vi "Edgertronic_SettingDialog.vi"(3 "URL":string="192.168.1.123") -> (1 "Saved Settings:":T4={"Requested Genlock "="20140911165611", "Min Frame Clocks "="20140911165611", "Is Seq Clk Freq "="20140911165611", "Pretrigger Frames "="20140911165611", "Duration "="20140911165611", "Overclock "="20140911165611", "Requested Horizontal "="20140911165611", "Frames "="20140911165611", "Requested Pretrigger "="20140911165611", "Words per Frame "="20140911165611", "Buffer End "="20140911165611", "Clocks per Frame  "="20140911165611", "Requested Duration "="20140911165611", "Pretrigger "="20140911165611", "Post-trigger Frames "="20140911165611", "Vertical "="20140911165611", "Requested Vertical "="20140911165611", "Reqested Frame Rate "="20140911165611", "Frame Rate "="20140911165611", "Horizontal "="20140911165611", "Clocks per Exposure "="20140911165611", "Digital Gain "="20140911165611", "Exposure "="20140911165611", "Genlock "="20140911165611", "Analog Gain "="20140911165611", "Subsample "="20140911165611", "Requested Exposure "="20140911165611", "Iso "="20140911165611", "Requested Overclock "="20140911165611", "Requested Subsample "="20140911165611", "Requested Iso"="20140911165611", "Multishot"="20140911165611", "Requested Multishot"="20140911165611", "Monochrome"="20140911165611", "Requested mono"="20140911165611", "FPGA Temp"="20140911165611", "Is Temp"="20140911165611", "Posttrigger Duration"="20140911165611", "Pretrigger Duration"="20140911165611", "dacvrefadc"="20140911165611"})   [LabVIEW 2015]
uses:
  GET/SettingsCtrl.ctl
panel:
  out "Image":picture
  in  "Settings":T1={"Frame Rate (fps)"=1000.0, "Exposure (1/sec)"=1500.0, "Horizonal"=0, "Vertical"=0, "ISO"=500, "Duration"=1.0, "Pretrigger (%)"=50.0, "MultiShot"=1, "Subsample?"=FALSE, "Force Mono?"=FALSE, "Genlock"=enum."Off", "Overclock"=enum."Off"} {"Pretrigger (%)" min=0.0 max=100.0 step=1.0 scale=0.0..100.0; "ISO" min=0 max=1600 step=1 scale=400.0..1600.0; "Vertical" scale=0.0..1024.0; "Horizonal" scale=0.0..1280.0; "Exposure (1/sec)" min=4e-06 max=250000.0 step=1.0 scale=10.0..250000.0; "Frame Rate (fps)" min=0.1 max=25000.0 step=1.0 scale=0.1..25000.0}
  in  "Controls":T2
  out "Camera Info":T3={"Hardware Build Date"=timestamp(3503952000 s since 1904-01-01), "Software Build Date"=timestamp(3493324800 s since 1904-01-01), "FPGA Initialized"="1", "Hardware Revision"="6", "Model"="1", "Home Dir"="/home/root/ss-web", "IR Filter"="1", "Mac Address"="00:1B:C5:09:61:4D", "Serial Console Enabled"="false", "Serial number"="333", "FPGA Version"="70", "Hardware Configuration"="1", "Connection Information:"="HTTP/1.0 200 OK\r\nContent-Type: text/html; charset=utf-8\r\nContent-Length: 313\r\nConnection: close\r\nDate: Tue, 14 Jun 2016 14:20:06 GMT\r\nServer: lighttpd/1.4.11 (edgertonic slow motion camera)"} {"Software Build Date" format="%<%x>T"; "Hardware Build Date" format="%<%x>T"}
  in  "Run":bool
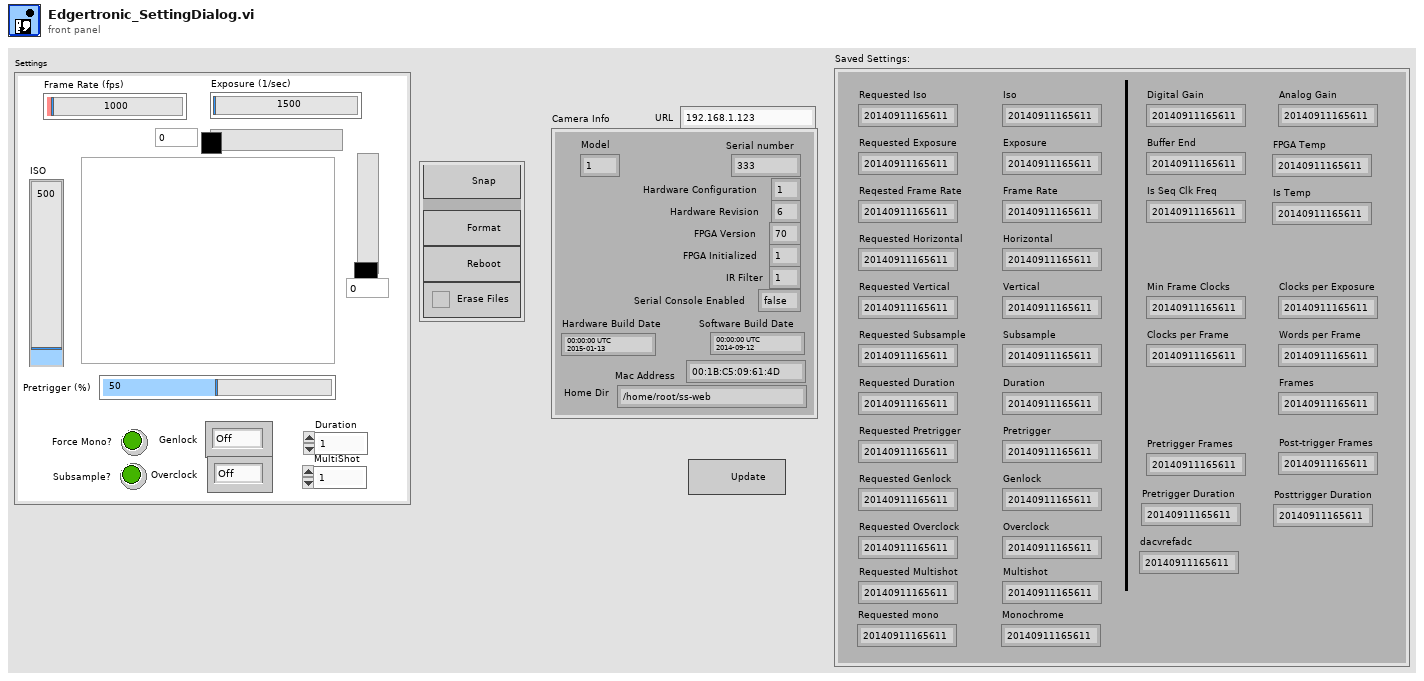
[diagram p1: front panel]
types:
  T1 = cluster{"Frame Rate (fps)":dbl, "Exposure (1/sec)":dbl, "Horizonal":u16, "Vertical":u16, "ISO":i16, "Duration":dbl, "Pretrigger (%)":dbl, "MultiShot":i16, "Subsample?":bool, "Force Mono?":bool, "Genlock":enum16{"Off", "Master", "Slave"}, "Overclock":enum16{"Off", "A level", "B Level", "C Level", "D Level"}}
  T2 = cluster{"Trigger":bool, "Cancel":bool, "Stop Save":bool, "Format":bool, "Reboot":bool, "Trash":bool}
  T3 = cluster{"Hardware Build Date":timestamp, "Software Build Date":timestamp, "FPGA Initialized":string, "Hardware Revision":string, "Model":string, "Home Dir":string, "IR Filter":string, "Mac Address":string, "Serial Console Enabled":string, "Serial number":string, "FPGA Version":string, "Hardware Configuration":string, "Connection Information:":string}
  T4 = typedef "SettingsCtrl.ctl" = cluster{"Requested Genlock ":string, "Min Frame Clocks ":string, "Is Seq Clk Freq ":string, "Pretrigger Frames ":string, "Duration ":string, "Overclock ":string, "Requested Horizontal ":string, "Frames ":string, "Requested Pretrigger ":string, "Words per Frame ":string, "Buffer End ":string, "Clocks per Frame  ":string, "Requested Duration ":string, "Pretrigger ":string, "Post-trigger Frames ":string, "Vertical ":string, "Requested Vertical ":string, "Reqested Frame Rate ":string, "Frame Rate ":string, "Horizontal ":string, "Clocks per Exposure ":string, "Digital Gain ":string, "Exposure ":string, "Genlock ":string, "Analog Gain ":string, "Subsample ":string, "Requested Exposure ":string, "Iso ":string, "Requested Overclock ":string, "Requested Subsample ":string, "Requested Iso":string, "Multishot":string, "Requested Multishot":string, "Monochrome":string, "Requested mono":string, "FPGA Temp":string, "Is Temp":string, "Posttrigger Duration":string, "Pretrigger Duration":string, "dacvrefadc":string}
  T5 = cluster{"Build Date":timestamp, "Software Build Date":timestamp, "FPGA Initialized":string, "Hardware Revision":string, "Model Number":string, "Home Dir":string, "IR Filter":string, "Mac Address":string, "Serial Console Enabled":string, "Serial number":string, "FPGA Version":string, "Hardware Configuration":string, "Connection Information:":string}
  T6 = typedef "imagedata.ctl" = cluster{"image type":i32, "image depth":i32, "image":u8[], "mask":u8[], "colors":u32[], "Rectangle":cluster{"left":i16, "top":i16, "right":i16, "bottom":i16}}
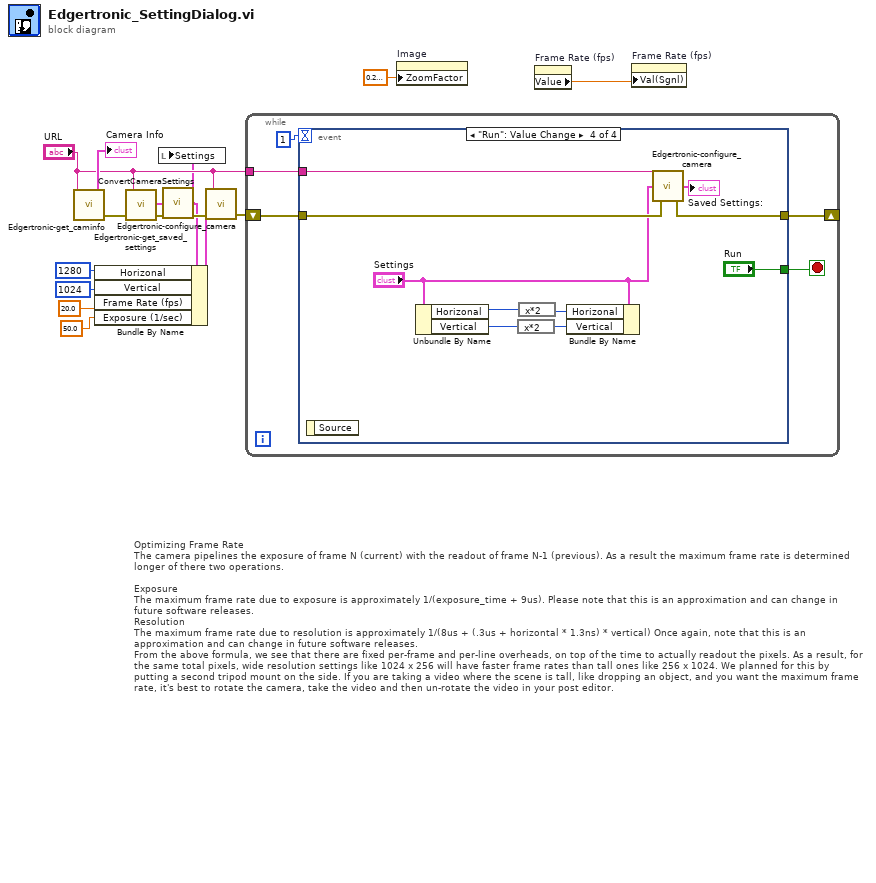
[diagram p0: block diagram]
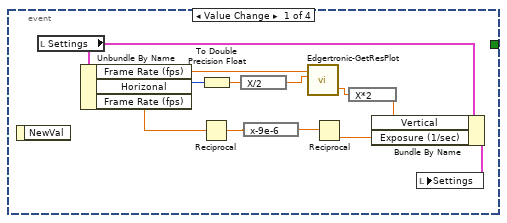
[diagram p2: hidden frame]
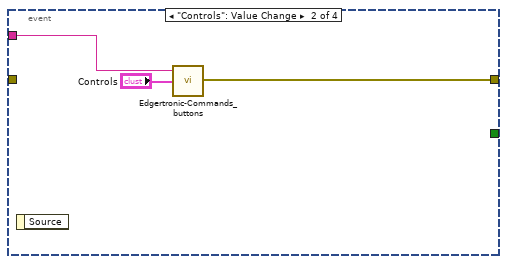
[diagram p3: hidden frame]
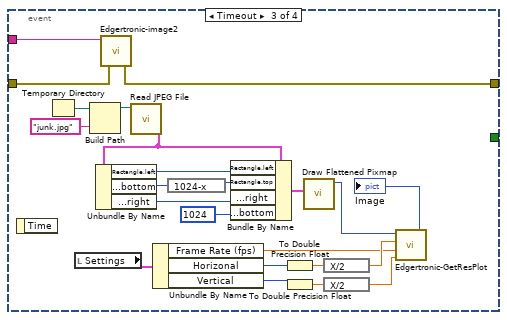
[diagram p4: hidden frame]
diagram:
  # "Optimizing Frame Rate\nThe camera pipelines the exposure of frame N (current) with the readout of frame N-1 (previous). As a result the maximum frame rate is determined longer of there two operations.\n\nExposure\nThe maximum frame rate due to exposure is approximately 1/(exposure_time + 9us). Please note that this is an approximation and can change in future software releases.\nResolution\nThe maximum frame rate due to resolution is approximately 1/(8us + (.3us + horizontal * 1.3ns) * vertical) Once again, note that this is an approximation and can change in future software releases.\nFrom the above formula, we see that there are fixed per-frame and per-line overheads, on top of the time to actually readout the pixels. As a result, for the same total pixels, wide resolution settings like 1024 x 256 will have faster frame rates than tall ones like 256 x 1024. We planned for this by putting a second tripod mount on the side. If you are taking a video where the scene is tall, like dropping an object, and you want the maximum frame rate, it's best to rotate the camera, take the video and then un-rotate the video in your post editor."
  n1 = call "Edgertronic-get_caminfo.vi"("URL"="URL") -> ("error out"=w11:errorcluster, "Cam Info"=→"Camera Info":T5)  [unwired: 3 in]
  n2 = call "Edgertronic-get_saved_settings.vi"("error in (no error)"=w11, "URL"="URL") -> ("error out"=w8:errorcluster, "Saved Settings:"=w10:T4)  [unwired: 2 in]
  n3 = call "ConvertCameraSettings.vi"("Saved Settings:"=w10) -> ("Settings"=w6:T1)
  n4 = Bundle By Name(cluster=w6, "Horizonal"=u16 1280, "Vertical"=u16 1024, "Frame Rate (fps)"=20.0, "Exposure (1/sec)"=50.0 ("Frame Rate (fps)")) -> (w3:T1)
  n5 = local write "Settings"(w6) -> ()
  n6 = call "Edgertronic-configure_camera.vi"("error in (no error)"=w8, "Settings"=w3, "URL"="URL") -> ("error out"=w7:errorcluster)  [unwired: 1 in, 1 out]
  n7 = while {
    tunnel: "URL" -> [w17]
    shift-right: [w15] -> _
    shift-left: w7 -> [w16]
    stop <- w19 stop-if-true
    n8 = event shown="[3] \"Run\": Value Change" {
      selector: _ -> [_ _ _ _]
      dyn-events: _ -> [_ _ _ _]
      timeout: 1 -> [_ _ _ _]
      tunnel: [_ _ _ "Run"] -> w19
      tunnel: w17 -> [_ w34 w57 w64]
      tunnel: [_ w32 w56 w62] -> w15
      tunnel: w16 -> [_ _ w45 w61]
      event "Settings.Horizonal", "Settings.Exposure (1/sec)", "Settings.Frame Rate (fps)": Value Change {
        n9 = event-data() -> ()  [unwired: 1 in, 1 out]
        n10 = local read "Settings"() -> (w23:T1)
        n11 = Unbundle By Name(w23) -> ("Frame Rate (fps)"=w25:dbl, "Horizonal"=w26:u16, "Frame Rate (fps)"=w24:dbl)
        n12 = Reciprocal(x=w24) -> (1/x=w30:dbl)
        n13 = To Double Precision Float(number=w26) -> (double precision float=w27:dbl)
        n14 = expression code="X/2"(w27) -> (w29:dbl)
        n15 = expression code="x-9e-6"(w30) -> (w31:dbl)
        n16 = call "Edgertronic-GetResPlot.vi"("Frame Rate (fps)"=w25, "Horizonal"=w29) -> ("Vertical"=w28:dbl)  [unwired: 2 in, 1 out]
        n17 = Reciprocal(x=w31) -> (1/x=w21:dbl)
        n18 = expression code="X*2"(w28) -> (w22:dbl)
        n19 = Bundle By Name(cluster=w23, "Vertical"=w22, "Exposure (1/sec)"=w21) -> (w20:T1)
        n20 = local write "Settings"(w20) -> ()
      }
      event "Controls": Value Change {
        n21 = event-data() -> ()  [unwired: 1 in, 1 out]
        n22 = call "Edgertronic-Commands_buttons.vi"("Controls"="Controls", "URL"=w34) -> ("error out"=w32:errorcluster)  [unwired: 2 in, 1 out]
      }
      event Timeout {
        n23 = event-data() -> ()  [unwired: 1 in, 1 out]
        n24 = Temporary Directory() -> (w55:path)
        n25 = local read "Settings"() -> (w41:T1)
        n26 = Build Path(base path=w55, name or relative path="junk.jpg") -> (appended path=w53:path)
        n27 = call "Edgertronic-image2.vi"("error in (no error)"=w45, "URL"=w57) -> ("error out"=w56:errorcluster)  [unwired: 1 in, 2 out]
        n28 = call <vilib>:"Read JPEG File.vi"("path to JPEG file"=w53) -> ("image data"=w52:T6)  [unwired: 8 in, 2 out]
        n29 = Unbundle By Name(w52) -> ("Rectangle.left"=w49:i16, "Rectangle.bottom"=w47:i16, "Rectangle.right"=w50:i16)
        n30 = Unbundle By Name(w41) -> ("Frame Rate (fps)"=w42:dbl, "Horizonal"=w43:u16, "Vertical"=w37:u16)
        n31 = expression code="1024-x"(w47) -> (w48:i16)
        n32 = Bundle By Name(cluster=w52, "Rectangle.left"=w49, "Rectangle.top"=w48, "Rectangle.right"=w50, "Rectangle.bottom"=1024) -> (w51:T6)
        n33 = To Double Precision Float(number=w43) -> (double precision float=w36:dbl)
        n34 = To Double Precision Float(number=w37) -> (double precision float=w38:dbl)
        n35 = call <vilib>:"Draw Flattened Pixmap.vi"("image data"=w51) -> ("new picture"=w40:picture)  [unwired: 8 in]
        n36 = expression code="X/2"(w36) -> (w44:dbl)
        n37 = expression code="X/2"(w38) -> (w35:dbl)
        n38 = call "Edgertronic-GetResPlot.vi"("Vertical"=w35, "Frame Rate (fps)"=w42, "Horizonal"=w44, "picture"=w40) -> ("2D Picture"=→"Image":picture)  [unwired: 1 out]
      }
      event "Run": Value Change {
        n39 = event-data() -> ()  [unwired: 1 in, 1 out]
        n40 = Unbundle By Name("Settings") -> ("Horizonal"=w60:u16, "Vertical"=w59:u16)
        n41 = expression code="x*2"(w59) -> (w66:u16)
        n42 = expression code="x*2"(w60) -> (w65:u16)
        n43 = Bundle By Name(cluster="Settings", "Horizonal"=w65, "Vertical"=w66) -> ()  [unwired: 1 out]
        n44 = call "Edgertronic-configure_camera.vi"("error in (no error)"=w61, "Settings"="Settings", "URL"=w64) -> ("error out"=w62:errorcluster, "Saved Settings:"=→"Saved Settings:":T4)  [unwired: 1 in]
      }
    }
  }
  n45 = property on="Image" class="Pict"("ZoomFactor"=sgl 0.2 ("Zoom Factor")) -> ()  [unwired: 2 in, 2 out]
  n46 = property on="Frame Rate (fps)" class="Slide (strict)"() -> ("Value"=w14:dbl)  [unwired: 2 in, 2 out]
  n47 = property on="Frame Rate (fps)" class="Slide (strict)"("Val(Sgnl)"=w14) -> ()  [unwired: 2 in, 2 out]
